vi "Set Param.vi"(8 "error in (no error)":errorcluster, 10 "param":dbl, 11 "paramID":i32) -> (0 "error out":errorcluster, 3 "function return":i32)   [LabVIEW 2020, in "ThorECU.lvlib"]
doc: "long SetParam(const long paramID, const double param);"
uses:
  ThorECU.lvlib
  ThorECU.dll
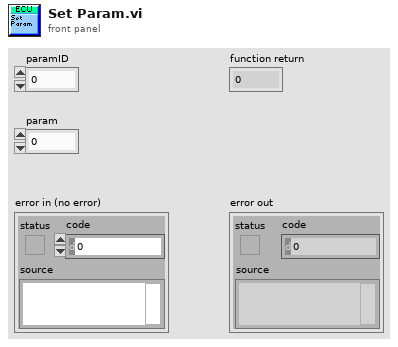
[diagram p1: front panel]
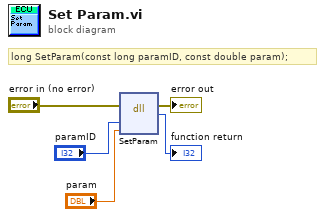
[diagram p0: block diagram]
diagram:
  # "long SetParam(const long paramID, const double param);"
  n1 = dll-call lib="D:/software/TweezerTron/ThorECU.*" fn="SetParam"(error in="error in (no error)", "paramID"="paramID", "param"="param") -> (error out=→"error out":errorcluster, "return type"=→"function return":i32)  [unwired: 4 in, 1 out]
